vi "ASCII Alphabet Letter.vi"(10 "Upper Case?":bool, 11 "Position in Alphabet":u32) -> (3 "Letter of Alphabet":string)   [LabVIEW 2014, in "Robot Actor Framework.lvlib" / "Utilities.lvlib"]
uses:
  Utilities.lvlib
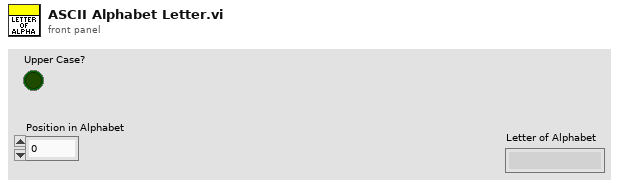
[diagram p1: front panel]
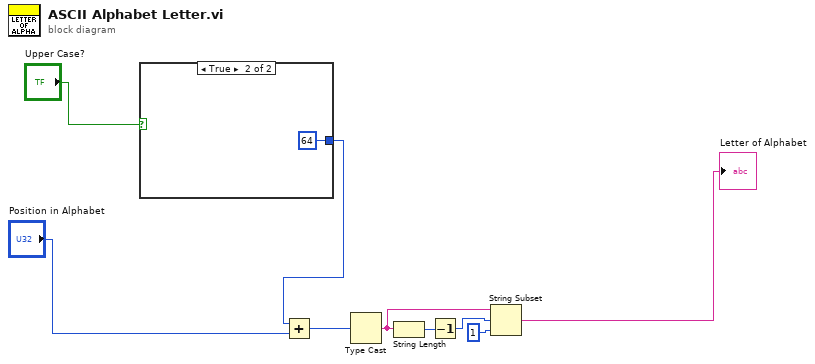
[diagram p0: block diagram]
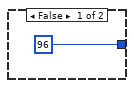
[diagram p2: hidden frame]
diagram:
  n1 = case shown="True" "Upper Case?" {
    tunnel: [96 64] -> w5
    frame False {
    }
    frame True {
    }
  }
  n2 = Add(x=w5, y="Position in Alphabet") -> (x+y=w6:u32)
  n3 = Type Cast(x=w6) -> (*(type *) &x=w2:string)  [unwired: 1 in]
  n4 = String Length(string=w2) -> (length=w8:i32)
  n5 = Decrement(x=w8) -> (x-1=w3:i32)
  n6 = String Subset(string=w2, offset (0)=w3, length (rest)=1 ("length (rest)")) -> (substring=→"Letter of Alphabet":string)
